vi "TriggerSetUp.vi"(2 "trigger holdoff (micsec)":dbl format="%.2f", 3 "trigger slope":i32(slide)=1, 4 "errorin":errorcluster, 5 "trigger level (volts)":dbl=0.2 format="%.2f", 6 "trigger source":string(combo)="VAL_EXTERNALxN", 7 "instrument handle in":refnum<k15>) -> (0 "error out":errorcluster, 1 "inst handle out":refnum<k15>)   [LabVIEW 2022 SP3]
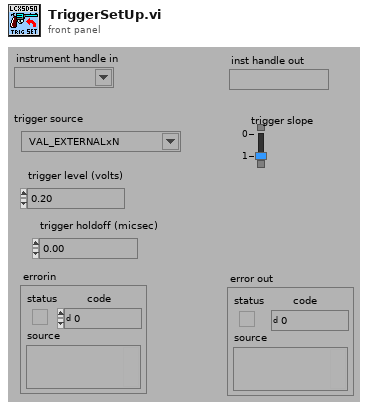
[diagram p1: front panel]
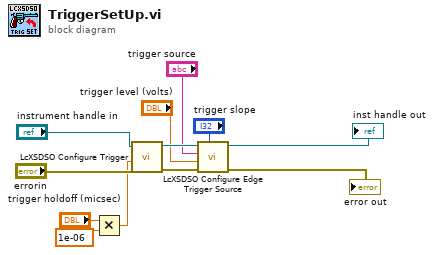
[diagram p0: block diagram]
diagram:
  n1 = Multiply(x="trigger holdoff (micsec)", y=1e-06) -> (x*y=w2:dbl)
  n2 = call "LcXSDSO Configure Trigger.vi"("error in (no error)"="errorin", "trigger holdoff (sec)"=w2, "instrument handle"="instrument handle in") -> ("error out"=w7:errorcluster, "instrument handle out"=w8:refnum<k15>)  [unwired: 7 in]
  n3 = call "LcXSDSO Configure Edge Trigger Source.vi"("trigger slope"="trigger slope", "error in (no error)"=w7, "trigger level (volts)"="trigger level (volts)", "trigger source"="trigger source", "instrument handle"=w8) -> ("error out"=→"error out":errorcluster, "instrument handle out"=→"inst handle out":refnum<k15>)  [unwired: 5 in]
